vi "AssertLessThan_Tests.vi"(11 "error in (no error)":errorcluster) -> (15 "error out":errorcluster)   [LabVIEW 2016, in "DronaTest.lvlib"]
uses:
  DronaTest.lvlib
  APIs/Assert/AssertControlValue/LessOrEqual.vi
  APIs/Assert/AssertControlValue/Less.vi
  <vilib>/addons/_JKI Toolkits/Caraya/classes/Assert/Assert Error.vi
  <vilib>/addons/_JKI Toolkits/Caraya/classes/Assert/Assert Less_Variant.vi
  <vilib>/addons/_JKI Toolkits/Caraya/classes/Assert/Assert Less Or Equal_Variant.vi
  <vilib>/addons/_JKI Toolkits/Caraya/classes/Test/Test.lvclass
  Drona.lvlib
  <vilib>/addons/_JKI Toolkits/Caraya/classes/Assert/Assert.lvclass
  APIs/Assert/AssertControlValue/AssertControlValue.lvlib
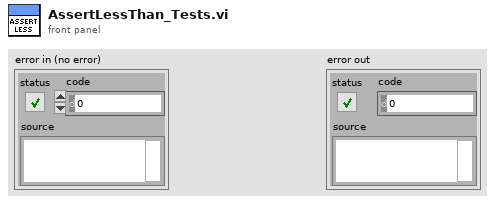
[diagram p1: front panel]
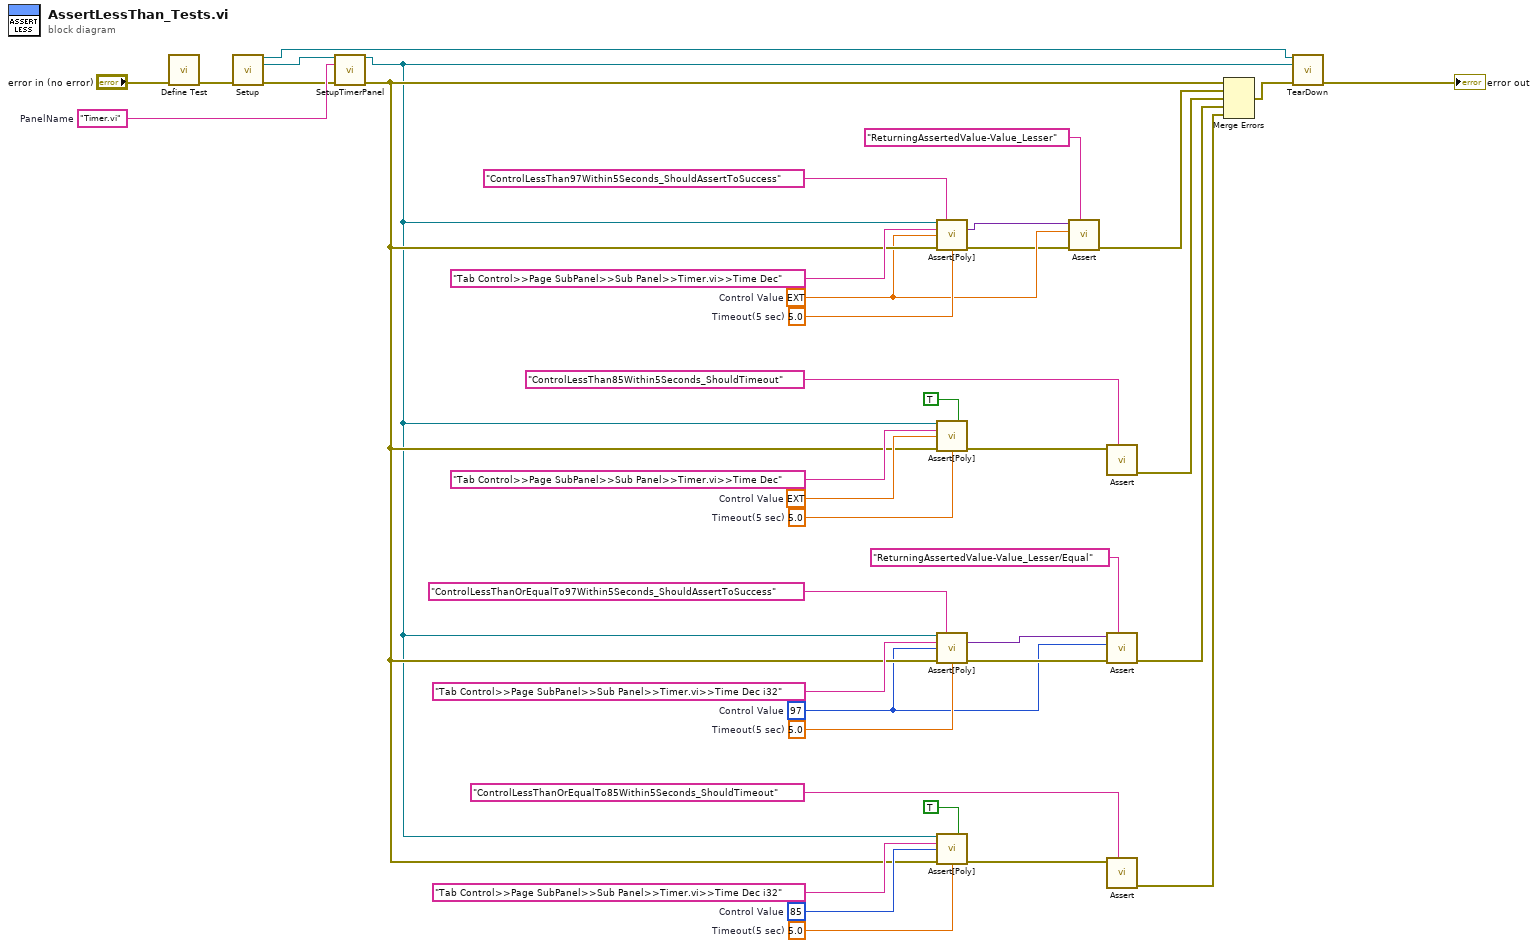
[diagram p0: block diagram]
diagram:
  w19 = "Timer.vi"  # PanelName
  w33 = 5.0  # Timeout(5 sec)
  w2 = 97  # Control Value
  w34 = 5.0  # Timeout(5 sec)
  w35 = 85  # Control Value
  w28 = 5.0  # Timeout(5 sec)
  w9 = ext 97.0  # Control Value
  w27 = 5.0  # Timeout(5 sec)
  w26 = ext 85.0  # Control Value
  n1 = call <vilib>:"Define Test.vi"("error in (no error)"="error in (no error)") -> ("error out"=w14:errorcluster)  [unwired: 10 in]
  n2 = call "Setup.vi"("error in (no error)"=w14) -> ("Application Ref"=w13:refnum<vi>, "VI out"=w17:refnum<vi>, "error out"=w18:errorcluster)  [unwired: 12 in]
  n3 = call "SetupTimerPanel.vi"("VI in"=w17, "Panel Name"=w19, "error in (no error)"=w18) -> ("VI out"=w11:refnum<vi>, "error out"=w12:errorcluster)  [unwired: 11 in]
  n4 = call-poly "Assert[Poly].vi"("VI Reference In"=w11, "Test Label"="ControlLessThan97Within5Seconds_ShouldAssertToSuccess" ("string"), "Control Path"="Tab Control>>Page SubPanel>>Sub Panel>>Timer.vi>>Time Dec", "Control Value"=w9, "Error In"=w12, "Timeout(5 sec)"=w28) -> ("Asserted Value"=w10:variant, "Error Out"=w8:errorcluster)  [unwired: 7 in, 1 out]
  n5 = call-poly "Assert[Poly].vi"("VI Reference In"=w11, "Assert Only? (F)"=TRUE, "Control Path"="Tab Control>>Page SubPanel>>Sub Panel>>Timer.vi>>Time Dec", "Control Value"=w26, "Error In"=w12, "Timeout(5 sec)"=w27) -> ("Error Out"=w24:errorcluster)  [unwired: 7 in, 2 out]
  n6 = call-poly "Assert[Poly].vi"("VI Reference In"=w11, "Test Label"="ControlLessThanOrEqualTo97Within5Seconds_ShouldAssertToSuccess" ("string"), "Control Path"="Tab Control>>Page SubPanel>>Sub Panel>>Timer.vi>>Time Dec i32", "Control Value"=w2, "Error In"=w12, "Timeout(5 sec)"=w33) -> ("Asserted Value"=w3:variant, "Error Out"=w5:errorcluster)  [unwired: 7 in, 1 out]
  n7 = call-poly "Assert[Poly].vi"("VI Reference In"=w11, "Assert Only? (F)"=TRUE, "Control Path"="Tab Control>>Page SubPanel>>Sub Panel>>Timer.vi>>Time Dec i32", "Control Value"=w35, "Error In"=w12, "Timeout(5 sec)"=w34) -> ("Error Out"=w37:errorcluster)  [unwired: 7 in, 2 out]
  n8 = call-poly <vilib>:"Assert.vi"("Label"="ReturningAssertedValue-Value_Lesser", "error in (no error)"=w8, "Y"=w9, "X"=w10) -> ("error out"=w7:errorcluster)  [unwired: 7 in]
  n9 = call-poly <vilib>:"Assert.vi"("Label"="ControlLessThan85Within5Seconds_ShouldTimeout" ("string"), "Error?"=w24) -> ("error out"=w21:errorcluster)  [unwired: 9 in]
  n10 = call-poly <vilib>:"Assert.vi"("Label"="ReturningAssertedValue-Value_Lesser/Equal", "error in (no error)"=w5, "Y"=w2, "X"=w3) -> ("error out"=w4:errorcluster)  [unwired: 7 in]
  n11 = call-poly <vilib>:"Assert.vi"("Label"="ControlLessThanOrEqualTo85Within5Seconds_ShouldTimeout" ("string"), "Error?"=w37) -> ("error out"=w20:errorcluster)  [unwired: 9 in]
  n12 = Merge Errors(w12, w7, w21, w4, w20) -> (w16:errorcluster)
  n13 = call "TearDown.vi"("Application Ref"=w13, "VI in"=w11, "error in (no error)"=w16) -> ("error out"=→"error out":errorcluster)  [unwired: 12 in]
